vi "Measurement Logic.vi"() -> ()   [LabVIEW 2021, in "Single Point_Channel Ganging.lvlib"]
uses:
  Single Point_Channel Ganging.lvlib
  Measurement Results.ctl
  <vilib>/Plug-In SDKs/Measurements/Measure Call Context/Measure Call Context.lvclass
  Measurement Configuration.ctl
  shared/Ganging/controls/Power ON-Ganging.ctl
  shared/Single/controls/Power ON-Single.ctl
panel:
  in  "measurement configuration":T1={"Mode of operation"=enum."Power on the DUT", "Source enable/disable"=TRUE, "Load enable/disable"=TRUE, "Power ON/Source resource names"=[], "Load resource names"=[], "Power ON/Source system configuration"=enum."Parallel", "Power ON/Source output function"=1006, "Power ON/Source voltage/current level"=6.0, "Source voltage/current level range"=20.0, "Power ON/Source sense"=1009, "Source limit symmetry"=enum."Asymmetric", "Power ON/Source current/voltage limit range"=25.0, "Source current/voltage limit low"=-0.6, "Source current/voltage limit high"=25.0, "Source transient response"=1038, "Source voltage gain bandwidth"=2000.0, "Source voltage compensation frequency"=3530.0, "Load device voltage/current rating"=30.0, "Source voltage pole-zero ratio"=2.0, "Load system configuration"=enum."Parallel", "Load output function"=1007, "Load voltage/current level"=2.0, "Load voltage/current level range"=40.0, "Load sense"=1009, "Load limit symmetry"=enum."Symmetric", "Load current/voltage limit range"=6.0, "Load current/voltage limit low"=0.0, "Load current/voltage limit high"=inf, "Load transient response"=1038, "Load current gain bandwidth"=14000.0, "Load current compensation frequency"=180000.0, "Load current pole-zero ratio"=0.3, "Aperture time"=0.01666, "Measurement duration"=1.0, "Measurement timeout"=1.0} {"Measurement timeout" format="%.3p"; "Load device voltage/current rating" format="%#_6pA"; "Load output function" items=["DC Voltage"=1006, "DC Current"=1007, "Pulse Voltage"=1049, "Pulse Current"=1050]; "Power ON/Source output function" items=["DC Voltage"=1006, "DC Current"=1007, "Pulse Voltage"=1049, "Pulse Current"=1050]; "Load sense" items=["Local"=1008, "Remote"=1009]; "Load transient response" items=["Slow"=1041, "Normal"=1038, "Fast"=1039, "Custom"=1042]; "Power ON/Source sense" items=["Local"=1008, "Remote"=1009]; "Source transient response" items=["Slow"=1041, "Normal"=1038, "Fast"=1039, "Custom"=1042]; "Measurement duration" format="%.3p"; "Aperture time" format="%.3p"; "Load current/voltage limit high" format="%#_6p"; "Load current/voltage limit low" format="%#_6p"; "Load current/voltage limit range" format="%#_6p"; "Load voltage/current level range" format="%#_6p"; "Load voltage/current level" format="%#_6p"; "Source current/voltage limit high" format="%#_6p"; "Source current/voltage limit low" format="%#_6p"; "Power ON/Source current/voltage limit range" format="%#_6p"; "Source voltage/current level range" format="%#_6p"; "Power ON/Source voltage/current level" format="%#_6p"}
  in  "error in":errorcluster
  out "measure call context out":refnum<class "Measure Call Context.lvclass">
  in  "measure call context in":refnum<class "Measure Call Context.lvclass">
  out "measurement results":T2
  out "error out":errorcluster
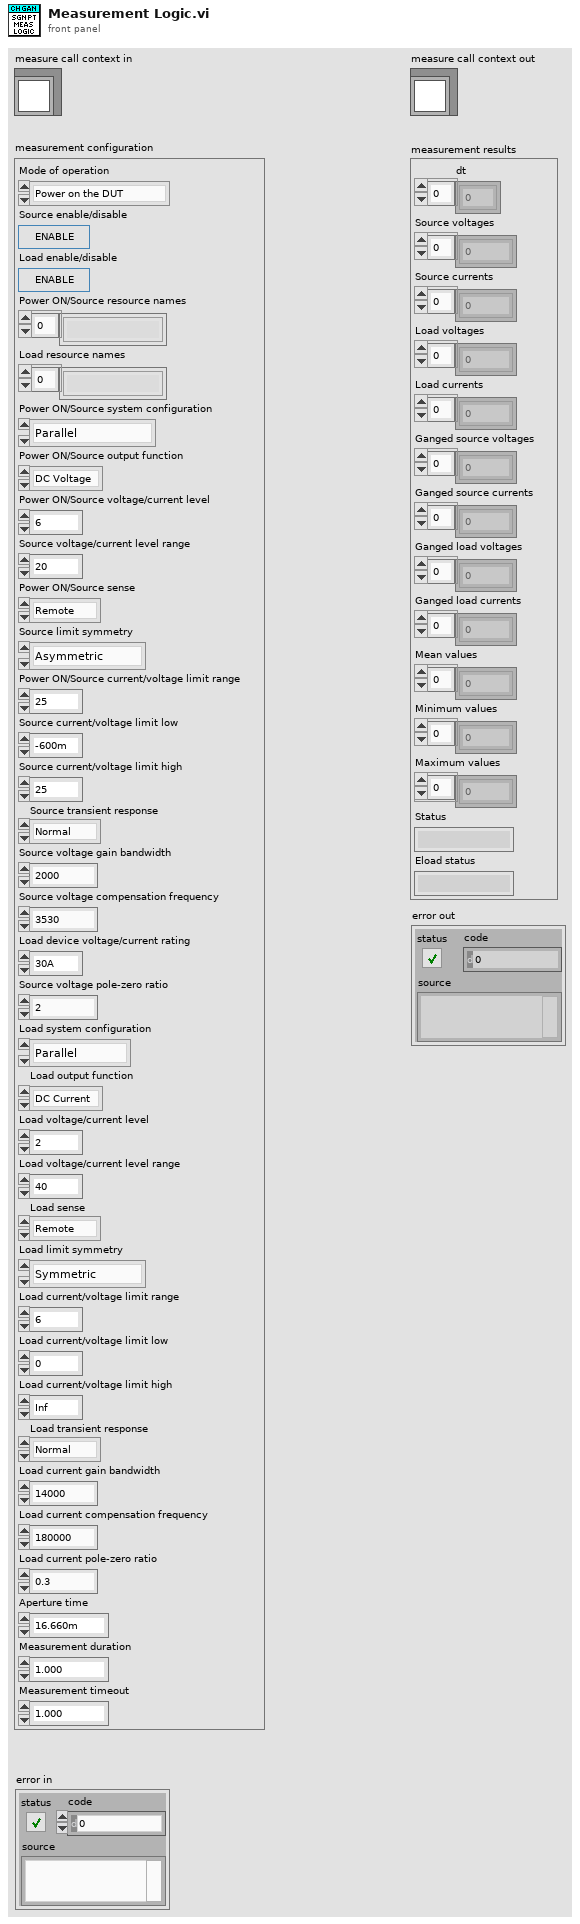
[diagram p1: front panel]
types:
  T1 = typedef "Single Point_Channel Ganging.lvlib/Measurement Configuration.ctl" = cluster{"Mode of operation":enum32{"Power on the DUT", "Perform measurement", "Power off the DUT"}, "Source enable/disable":bool, "Load enable/disable":bool, "Power ON/Source resource names":string[], "Load resource names":string[], "Power ON/Source system configuration":enum32{"Series", "Parallel", "Manual"}, "Power ON/Source output function":i32, "Power ON/Source voltage/current level":dbl, "Source voltage/current level range":dbl, "Power ON/Source sense":i32, "Source limit symmetry":enum32{"Symmetric", "Asymmetric"}, "Power ON/Source current/voltage limit range":dbl, "Source current/voltage limit low":dbl, "Source current/voltage limit high":dbl, "Source transient response":i32, "Source voltage gain bandwidth":dbl, "Source voltage compensation frequency":dbl, "Load device voltage/current rating":dbl, "Source voltage pole-zero ratio":dbl, "Load system configuration":enum32{"Series", "Parallel", "Manual"}, "Load output function":i32, "Load voltage/current level":dbl, "Load voltage/current level range":dbl, "Load sense":i32, "Load limit symmetry":enum32{"Symmetric", "Asymmetric"}, "Load current/voltage limit range":dbl, "Load current/voltage limit low":dbl, "Load current/voltage limit high":dbl, "Load transient response":i32, "Load current gain bandwidth":dbl, "Load current compensation frequency":dbl, "Load current pole-zero ratio":dbl, "Aperture time":dbl, "Measurement duration":dbl, "Measurement timeout":dbl}
  T2 = typedef "Single Point_Channel Ganging.lvlib/Measurement Results.ctl" = cluster{"dt":dbl[], "Source voltages":dbl[], "Source currents":dbl[], "Load voltages":dbl[], "Load currents":dbl[], "Ganged source voltages":dbl[], "Ganged source currents":dbl[], "Ganged load voltages":dbl[], "Ganged load currents":dbl[], "Mean values":dbl[], "Minimum values":dbl[], "Maximum values":dbl[], "Status":string, "Eload status":string}
  T3 = enum32{"Power on the DUT", "Perform measurement", "Power off the DUT"}
  T4 = typedef "Power ON-Ganging.ctl" = cluster{"Master/single Resource name":string, "Slave resource name":string[], "System configuration":enum32{"Series", "Parallel", "Manual"}, "Output function":i32, "Voltage/current level":dbl, "Voltage/current limit":dbl, "Sense":i32}
  T5 = typedef "Power ON-Single.ctl" = cluster{"Voltage/current level":dbl, "Voltage/current limit":dbl, "Sense":i32, "Resource name":string, "Output function":i32}
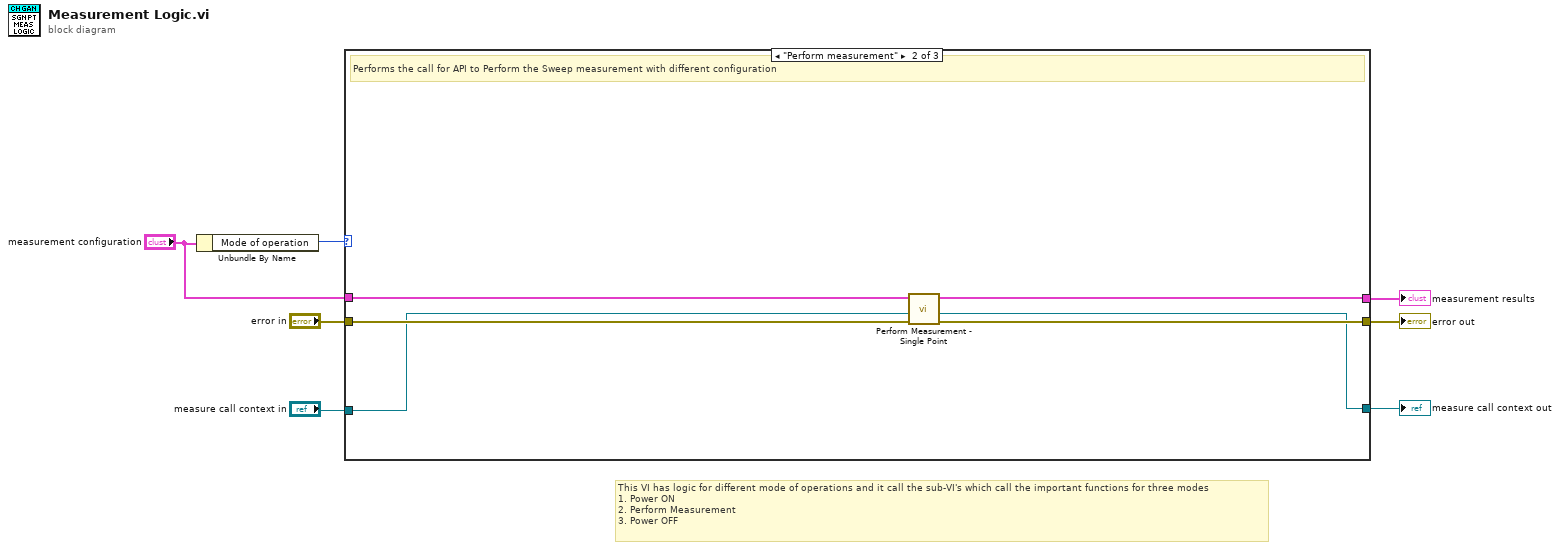
[diagram p0: block diagram]
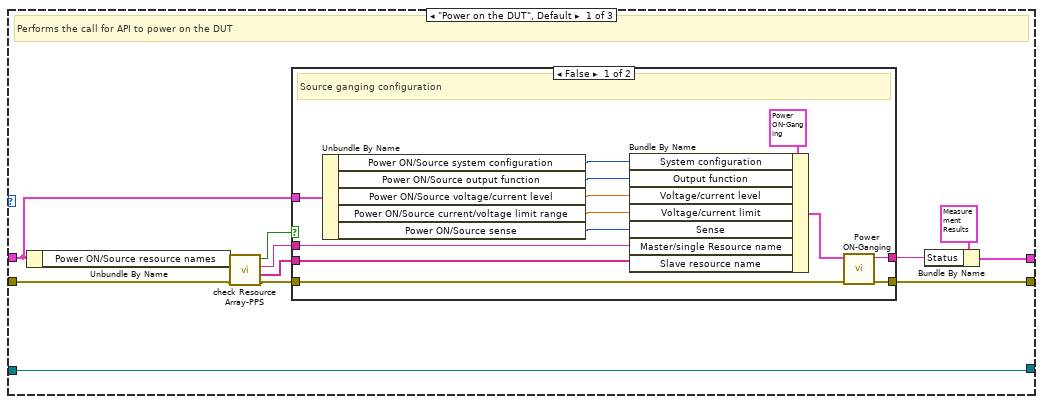
[diagram p2: hidden frame]
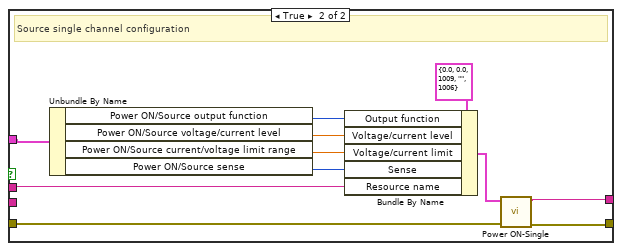
[diagram p3: hidden frame]
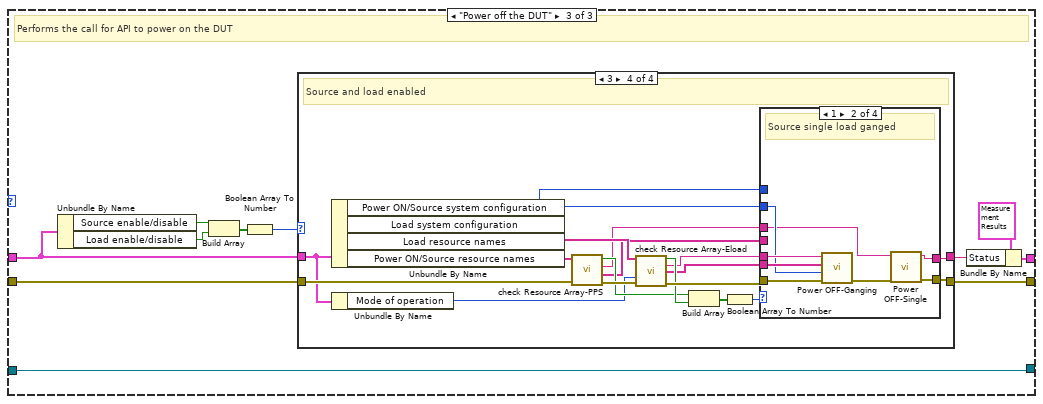
[diagram p4: hidden frame]
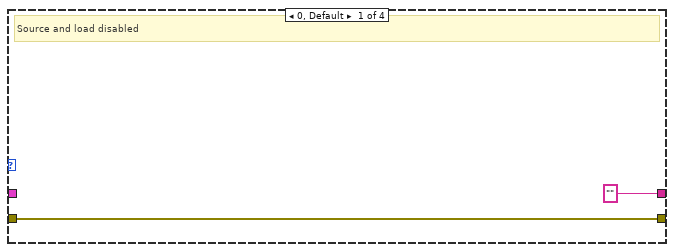
[diagram p5: hidden frame]
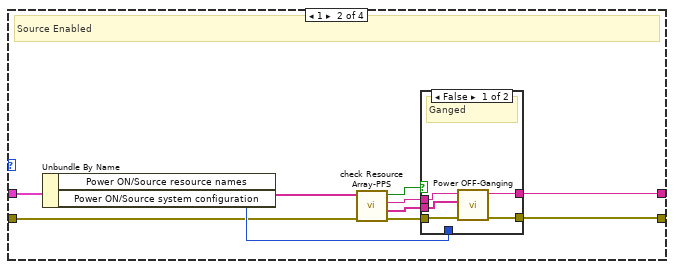
[diagram p6: hidden frame]
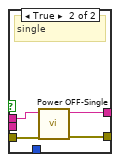
[diagram p7: hidden frame]
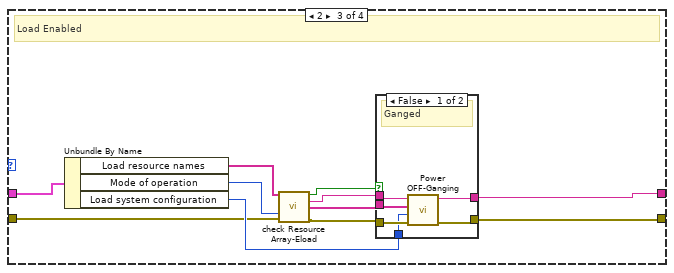
[diagram p8: hidden frame]
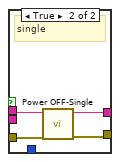
[diagram p9: hidden frame]
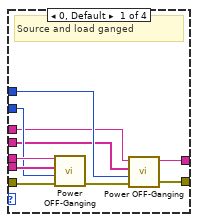
[diagram p10: hidden frame]
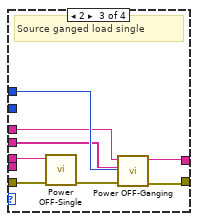
[diagram p11: hidden frame]
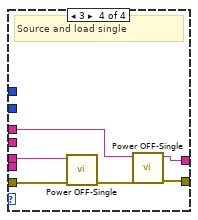
[diagram p12: hidden frame]
diagram:
  # "This VI has logic for different mode of operations and it call the sub-VI's which call the important functions for three modes\n1. Power ON\n2. Perform Measurement\n3. Power OFF"
  n1 = Unbundle By Name("measurement configuration") -> ("Mode of operation"=w7:T3)
  n2 = case shown="\"Perform measurement\"" w7 {
    tunnel: "error in" -> [w14 w49 w54]
    tunnel: [w13 w48 w53] -> w5
    tunnel: "measure call context in" -> [w12 w44 w50]
    tunnel: [w12 w47 w50] -> w3
    tunnel: "measurement configuration" -> [w11 w45 w55]
    tunnel: [w8 w46 w51] -> w2
    frame "Power on the DUT", Default {
      # "Performs the call for API to power on the DUT"
      n3 = Unbundle By Name(w11) -> ("Power ON/Source resource names"=w16:string[])
      n4 = call "check Resource Array-PPS.vi"("error in"=w14, "Resource names"=w16) -> ("error out"=w19:errorcluster, "Slave resource names"=w17:string[], "Single/Master resouce names"=w18:string, "Single or ganged configuration"=w15:bool)  [unwired: 6 in]
      n5 = case shown="False" w15 {
        tunnel: w19 -> [w24 w39]
        tunnel: [w25 w38] -> w13
        tunnel: w17 -> [w30 _]
        tunnel: w11 -> [w32 w43]
        tunnel: w18 -> [w31 w34]
        tunnel: [w26 w37] -> w9
        frame False {
          # "Source ganging configuration"
          n6 = Unbundle By Name(w32) -> ("Power ON/Source system configuration"=w23:enum32{"Series", "Parallel", "Manual"}, "Power ON/Source output function"=w22:i32, "Power ON/Source voltage/current level"=w29:dbl, "Power ON/Source current/voltage limit range"=w28:dbl, "Power ON/Source sense"=w27:i32)
          n7 = Bundle By Name(cluster=T4 {"Master/single Resource name"="", "Slave resource name"=[], "System configuration"=enum."Parallel", "Output function"=1006, "Voltage/current level"=0.0, "Voltage/current limit"=0.0, "Sense"=1009} ("Power ON"), "System configuration"=w23, "Output function"=w22, "Voltage/current level"=w29, "Voltage/current limit"=w28, "Sense"=w27, "Master/single Resource name"=w31, "Slave resource name"=w30) -> (w20:T4)
          n8 = call "Power ON-Ganging.vi"("error in"=w24, "Power ON"=w20) -> ("error out"=w25:errorcluster, "Status"=w26:string)  [unwired: 8 in]
        }
        frame True {
          # "Source single channel configuration"
          n9 = Unbundle By Name(w43) -> ("Power ON/Source output function"=w36:i32, "Power ON/Source voltage/current level"=w40:dbl, "Power ON/Source current/voltage limit range"=w41:dbl, "Power ON/Source sense"=w42:i32)
          n10 = Bundle By Name(cluster=T5 {"Voltage/current level"=0.0, "Voltage/current limit"=0.0, "Sense"=1009, "Resource name"="", "Output function"=1006} ("Power ON single"), "Output function"=w36, "Voltage/current level"=w40, "Voltage/current limit"=w41, "Sense"=w42, "Resource name"=w34) -> (w35:T5)
          n11 = call "Power ON-Single.vi"("error in"=w39, "Power ON single"=w35) -> ("error out"=w38:errorcluster, "Status"=w37:string)  [unwired: 8 in]
        }
      }
      n12 = Bundle By Name(cluster=T2 {"dt"=[], "Source voltages"=[], "Source currents"=[], "Load voltages"=[], "Load currents"=[], "Ganged source voltages"=[], "Ganged source currents"=[], "Ganged load voltages"=[], "Ganged load currents"=[], "Mean values"=[], "Minimum values"=[], "Maximum values"=[], "Status"="", "Eload status"=""} ("measurement results"), "Status"=w9) -> (w8:T2)
    }
    frame "Perform measurement" {
      # "Performs the call for API to Perform the Sweep measurement with different configuration"
      n13 = call "Perform Measurement - Single Point.vi"("error in (no error)"=w49, "Measure Call Context in"=w44, "measurement configuration"=w45) -> ("error out"=w48:errorcluster, "Measure Call Context out"=w47:refnum<class "Measure Call Context.lvclass">, "Measurement Results"=w46:T2)  [unwired: 6 in]
    }
    frame "Power off the DUT" {
      # "Performs the call for API to power on the DUT"
      n14 = Unbundle By Name(w55) -> ("Source enable/disable"=w60:bool, "Load enable/disable"=w59:bool)
      n15 = Build Array(w60, w59) -> (w58:bool[])
      n16 = Boolean Array To Number(Boolean array=w58) -> (number=w57:u32)
      n17 = case shown="3" w57 {
        tunnel: w55 -> [_ w72 w92 w104]
        tunnel: w54 -> [w62 w67 w88 w110]
        tunnel: [w62 w71 w91 w119] -> w53
        tunnel: ["" ("Status") w69 w90 w118] -> w56
        frame 0, Default {
          # "Source and load disabled"
        }
        frame 1 {
          # "Source Enabled"
          n18 = Unbundle By Name(w72) -> ("Power ON/Source resource names"=w68:string[], "Power ON/Source system configuration"=w70:enum32{"Series", "Parallel", "Manual"})
          n19 = call "check Resource Array-PPS.vi"("error in"=w67, "Resource names"=w68) -> ("error out"=w66:errorcluster, "Slave resource names"=w63:string[], "Single/Master resouce names"=w64:string, "Single or ganged configuration"=w65:bool)  [unwired: 6 in]
          n20 = case shown="False" w65 {
            tunnel: w66 -> [w77 w79]
            tunnel: [w73 w80] -> w71
            tunnel: [w76 w81] -> w69
            tunnel: w70 -> [_ _]
            tunnel: w64 -> [w75 w78]
            tunnel: w63 -> [w74 _]
            frame False {
              # "Ganged"
              n21 = call "Power OFF-Ganging.vi"("error in"=w77, "Slave resource names"=w74, "Master resouce name"=w75) -> ("error out"=w73:errorcluster, "Status"=w76:string)  [unwired: 7 in]
            }
            frame True {
              # "single"
              n22 = call "Power OFF-Single.vi"("error in (no error)"=w79, "Resource name"=w78) -> ("error out"=w80:errorcluster, "Status"=w81:string)  [unwired: 8 in]
            }
          }
        }
        frame 2 {
          # "Load Enabled"
          n23 = Unbundle By Name(w92) -> ("Load resource names"=w83:string[], "Mode of operation"=w82:T3, "Load system configuration"=w89:enum32{"Series", "Parallel", "Manual"})
          n24 = call "check Resource Array-Eload.vi"("Resource names"=w83, "Mode of operation"=w82, "error in"=w88) -> ("Single or ganged configuration"=w86:bool, "Single/Master resouce name"=w85:string, "Slave resource names"=w84:string[], "error out"=w87:errorcluster)  [unwired: 8 in, 1 out]
          n25 = case shown="False" w86 {
            tunnel: w87 -> [w98 w101]
            tunnel: [w93 w99] -> w91
            tunnel: [w97 w100] -> w90
            tunnel: w85 -> [w96 w102]
            tunnel: w84 -> [w95 _]
            tunnel: w89 -> [w94 _]
            frame False {
              # "Ganged"
              n26 = call "Power OFF-Ganging.vi"("error in"=w98, "Ganged Config"=w94, "Slave resource names"=w95, "Master resouce name"=w96) -> ("error out"=w93:errorcluster, "Status"=w97:string)  [unwired: 6 in]
            }
            frame True {
              # "single"
              n27 = call "Power OFF-Single.vi"("error in (no error)"=w101, "Resource name"=w102) -> ("error out"=w99:errorcluster, "Status"=w100:string)  [unwired: 8 in]
            }
          }
        }
        frame 3 {
          # "Source and load enabled"
          n28 = Unbundle By Name(w104) -> ("Power ON/Source system configuration"=w116:enum32{"Series", "Parallel", "Manual"}, "Load system configuration"=w117:enum32{"Series", "Parallel", "Manual"}, "Load resource names"=w111:string[], "Power ON/Source resource names"=w108:string[])
          n29 = Unbundle By Name(w104) -> ("Mode of operation"=w103:T3)
          n30 = call "check Resource Array-PPS.vi"("error in"=w110, "Resource names"=w108) -> ("error out"=w109:errorcluster, "Slave resource names"=w105:string[], "Single/Master resouce names"=w106:string, "Single or ganged configuration"=w107:bool)  [unwired: 6 in]
          n31 = call "check Resource Array-Eload.vi"("Resource names"=w111, "Mode of operation"=w103, "error in"=w109) -> ("Single or ganged configuration"=w114:bool, "Single/Master resouce name"=w113:string, "Slave resource names"=w112:string[], "error out"=w115:errorcluster)  [unwired: 8 in, 1 out]
          n32 = Build Array(w107, w114) -> (w121:bool[])
          n33 = Boolean Array To Number(Boolean array=w121) -> (number=w120:u32)
          n34 = case shown="1" w120 {
            tunnel: w115 -> [w130 w139 w147 w153]
            tunnel: [w122 w137 w140 w151] -> w119
            tunnel: [w131 w138 w143 w149] -> w118
            tunnel: w113 -> [w129 w136 w146 w150]
            tunnel: w112 -> [w128 w135 _ _]
            tunnel: w117 -> [w127 w134 _ _]
            tunnel: w116 -> [w126 _ w144 _]
            tunnel: w106 -> [w124 w133 w142 w148]
            tunnel: w105 -> [w125 _ w141 _]
            frame 0, Default {
              # "Source and load ganged"
              n35 = call "Power OFF-Ganging.vi"("error in"=w130, "Ganged Config"=w127, "Slave resource names"=w128, "Master resouce name"=w129) -> ("error out"=w123:errorcluster)  [unwired: 6 in, 1 out]
              n36 = call "Power OFF-Ganging.vi"("error in"=w123, "Ganged Config"=w126, "Slave resource names"=w125, "Master resouce name"=w124) -> ("error out"=w122:errorcluster, "Status"=w131:string)  [unwired: 6 in]
            }
            frame 1 {
              # "Source single load ganged"
              n37 = call "Power OFF-Ganging.vi"("error in"=w139, "Ganged Config"=w134, "Slave resource names"=w135, "Master resouce name"=w136) -> ("error out"=w132:errorcluster)  [unwired: 6 in, 1 out]
              n38 = call "Power OFF-Single.vi"("error in (no error)"=w132, "Resource name"=w133) -> ("error out"=w137:errorcluster, "Status"=w138:string)  [unwired: 8 in]
            }
            frame 2 {
              # "Source ganged load single"
              n39 = call "Power OFF-Single.vi"("error in (no error)"=w147, "Resource name"=w146) -> ("error out"=w145:errorcluster)  [unwired: 8 in, 1 out]
              n40 = call "Power OFF-Ganging.vi"("error in"=w145, "Ganged Config"=w144, "Slave resource names"=w141, "Master resouce name"=w142) -> ("error out"=w140:errorcluster, "Status"=w143:string)  [unwired: 6 in]
            }
            frame 3 {
              # "Source and load single"
              n41 = call "Power OFF-Single.vi"("error in (no error)"=w153, "Resource name"=w150) -> ("error out"=w152:errorcluster)  [unwired: 8 in, 1 out]
              n42 = call "Power OFF-Single.vi"("error in (no error)"=w152, "Resource name"=w148) -> ("error out"=w151:errorcluster, "Status"=w149:string)  [unwired: 8 in]
            }
          }
        }
      }
      n43 = Bundle By Name(cluster=T2 {"dt"=[], "Source voltages"=[], "Source currents"=[], "Load voltages"=[], "Load currents"=[], "Ganged source voltages"=[], "Ganged source currents"=[], "Ganged load voltages"=[], "Ganged load currents"=[], "Mean values"=[], "Minimum values"=[], "Maximum values"=[], "Status"="", "Eload status"=""} ("measurement results"), "Status"=w56) -> (w51:T2)
    }
  }
  "error out" <- w5
  "measurement results" <- w2
  "measure call context out" <- w3
